vi "Preview_Build.vi"(8 "error in (no error)":errorcluster, 11 "Build in":refnum<class "AB_WebService.lvclass">) -> (0 "error out":errorcluster, 1 "GeneratedFiles":path[](array[path]), 3 "Build out":refnum<class "AB_WebService.lvclass">, 4 "GeneratedFileGUIDs":string[](array[string]), 5 "OutputDirectory":path)   [LabVIEW 2020, in "AB_WebService.lvclass"]
uses:
  <vilib>/AppBuilder/AB_Classes/WebService/AB_WebService.lvclass
  <vilib>/AppBuilder/AB_Classes/WebService/AB_WebService.lvclass/AB_WebService.ctl
  <vilib>/AppBuilder/AB_Classes/Build/AB_Build.lvclass
  <vilib>/AppBuilder/AB_Classes/TargetFile/AB_Targetfile.lvclass
  e:/builds/penguin/labview/branches/2020/dev/dist/vi.lib/AppBuilder/AB_Classes/TargetFile/AB_Targetfile.lvclass
  e:/builds/penguin/labview/branches/2020/dev/dist/vi.lib/AppBuilder/AB_Classes/Build/AB_Build.lvclass
  e:/builds/penguin/labview/branches/2020/dev/dist/vi.lib/AppBuilder/AB_Classes/WebService/AB_WebService.lvclass
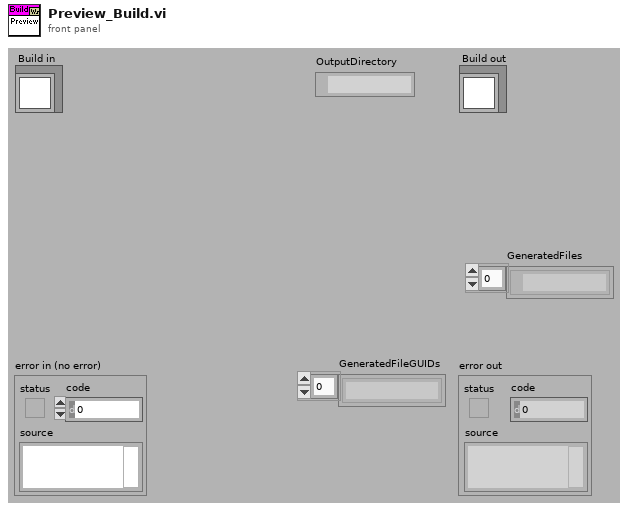
[diagram p1: front panel]
types:
  T1 = typedef "AB_Build.ctl" = cluster{"buildSpecName":string, "buildSpecDescription":string, "destinations":refnum<class "AB_Destination.lvclass">[], "exclusionOption":T2, "defaultLanguage":string, "supportedLanguages":string[], "excludedDirectories":path[], "buildContext":refnum<vi>, "buildObject":T3, "preview":bool, "programatic":bool, "progressBarEvents":T4, "userLog_Path":path, "preActionID":string, "preAction_Path":path, "postActionID":string, "postAction_Path":path, "eng_checkForBrokenVIs?":bool, "eng_verboseLinkerErrors?":bool, "localDest_Path":path, "targetDest_Path":path, "removeVIObject":u16, "cache":refnum<class "PreviewCache.lvclass">, "use cache":bool, "previewCache_ID":string, "buildCache_ID":string, "eng_TempLocalDest_Path":path, "eng_collectDependencies?":bool, "versionInfo":cluster{"buildVersion":cluster{"major":u16, "minor":u16, "patch":u16, "build":u16}, "autoIncrement":bool}, "eng_enableVIChecksums":bool}
  T2 = typedef "AB_Exclusion_Option.ctl" = cluster{"typedefs":bool, "polymorphicVIs":bool, "unusedLibraryItems":bool, "modifyLibraryFile":bool, "edit-timeDependencies":bool, "inlineVIs":bool, "dependent PPLs":bool, "dependent DLLs":bool}
  T3 = typedef "ItemRef.ctl" = u64
  T4 = typedef "provcom_ProgressBar_Events.ctl" = cluster{"newJob":refnum<user-event>, "newItem":refnum<user-event>, "errorMsg":T5, "cancel":refnum<user-event>}
  T5 = typedef "mxLvBuildError.ctl" = refnum<user-event>
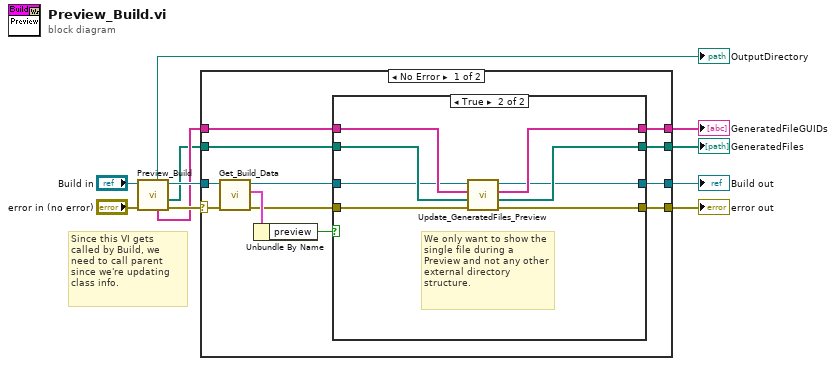
[diagram p0: block diagram]
diagram:
  # "Since this VI gets called by Build, we need to call parent since we're updating class info."
  n1 = call-parent "Preview_Build.vi"("error in (no error)"="error in (no error)", "Build in"="Build in") -> ("error out"=w8:errorcluster, "GeneratedFiles"=w3:path[], "Build out"=w6:refnum<class "AB_WebService.lvclass">, "GeneratedFileGUIDs"=w4:string[], "OutputDirectory"=→"OutputDirectory":path)  [unwired: 5 out]
  n2 = case shown="No Error" w8 {
    selector: w8 -> [w21 w38]
    tunnel: [w13 w38] -> w7
    tunnel: w6 -> [w22 w39]
    tunnel: [w12 w39] -> w5
    tunnel: w4 -> [w19 w36]
    tunnel: w3 -> [w20 w37]
    tunnel: [w16 w37] -> w2
    tunnel: [w17 w36] -> w1
    frame No Error {
      n3 = call <vilib>:"Get_Build_Data.vi"("error in (no error)"=w21, "Class in"=w22) -> ("error out"=w15:errorcluster, "data"=w23:T1, "Class out"=w18:refnum<class "AB_WebService.lvclass">)  [unwired: 7 out]
      n4 = Unbundle By Name(w23) -> ("preview"=w14:bool)
      n5 = case shown="True" w14 {
        tunnel: w20 -> [w26 w34]
        tunnel: w19 -> [w27 w35]
        tunnel: w18 -> [w25 w31]
        tunnel: [w27 w33] -> w17
        tunnel: [w26 w32] -> w16
        tunnel: w15 -> [w24 w29]
        tunnel: [w24 w28] -> w13
        tunnel: [w25 w30] -> w12
        frame False {
          # "When building, we need the generated files to be the actual files that will be created so don't modify array."
        }
        frame True {
          # "We only want to show the single file during a Preview and not any other external directory structure."
          n6 = call-dynamic "Update_GeneratedFiles_Preview.vi"("error in (no error)"=w29, "GeneratedFiles in"=w34, "GeneratedFileGUIDs in"=w35, "Build in"=w31) -> ("error out"=w28:errorcluster, "GeneratedFiles out"=w32:path[], "GeneratedFileGUIDs out"=w33:string[], "Build out"=w30:refnum<class "AB_WebService.lvclass">)  [unwired: 4 in]
        }
      }
    }
    frame Error {
    }
  }
  "error out" <- w7
  "Build out" <- w5
  "GeneratedFiles" <- w2
  "GeneratedFileGUIDs" <- w1
